vi "GetAngleBetweenPoints.vi"(0 "x0":dbl, 5 "y0":dbl, 9 "x1":dbl, 11 "y1":dbl, 12 "x2":dbl, 13 "y2":dbl) -> (8 "angle":dbl)   [LabVIEW 2012]
uses:
  <vilib>/imath/engines/lvmath2/RunTimeEngine/BuiltInFunctions/atan2/NIMS_atan2.vi
  <instcachedir>/0/NIMS_atan2_A91AA4A7D42247EDBE8F76DB99AF04A4.lvgen/NIMS_atan2_A91AA4A7D42247EDBE8F76DB99AF04A4_000.vi
  <vilib>/imath/engines/lvmath2/RunTimeEngine/NodeEndStatement/NIMS_NodeEndStatement_Output.vi
  <instcachedir>/0/NIMS_NodeEndStatement_Output_53EC0D466D134D7ABD903AC30B43404B.lvgen/NIMS_NodeEndStatement_Output_53EC0D466D134D7ABD903AC30B43404B_001.vi
  <vilib>/imath/engines/lvmath2/RunTimeEngine/ErrorHandling/NIMS_Finalize Error.vi
panel:
  out "theta2":dbl
  out "theta0":dbl
  # "origin"
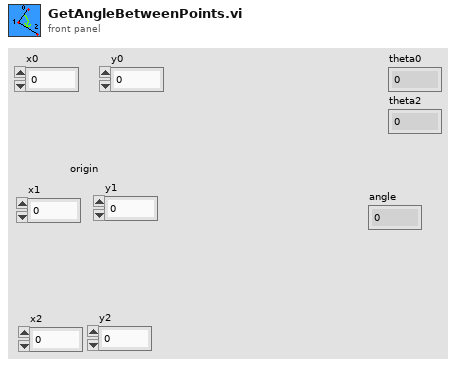
[diagram p1: front panel]
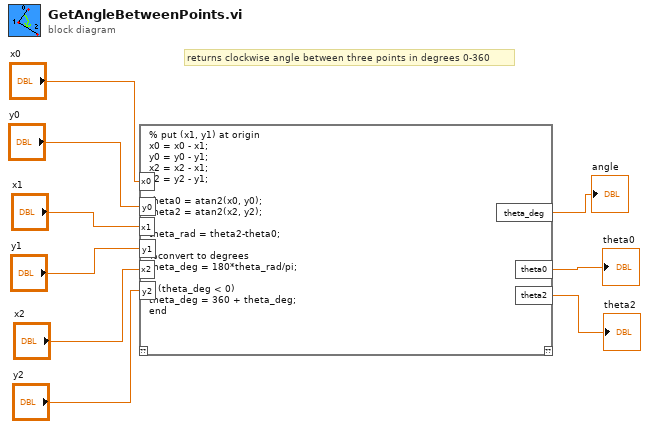
[diagram p0: block diagram]
diagram:
  # "returns clockwise angle between three points in degrees 0-360"
  n1 = mathscript code="% put (x1, y1) at origin\nx0 = x0 - x1;\ny0 = y0 - y1;\nx2 = x2 - x1;\ny2 = y2 - y1;\n\ntheta0 = atan2(x0, y0);\ntheta2 = atan2(x2, y2);\n\ntheta_rad = theta2-theta0;\n\n%convert to degrees\ntheta_deg = 180*theta_rad/pi;\n\nif (theta_deg < 0)\ntheta_deg = 360 + theta_deg;\nend"("x0"="x0", "y0"="y0", "x1"="x1", "y1"="y1", "x2"="x2", "y2"="y2") -> ("theta_deg"=→"angle":dbl, "theta0"=→"theta0":dbl, "theta2"=→"theta2":dbl)  [unwired: 1 in, 1 out]
